vi "RT Main system.vi"   [LabVIEW 2018]
uses:
  <vilib>/FPGAPlugInAG/myRIO-1900/niLvFpga_Open_myRIO-1900.vi
  <vilib>/rvi/interface/common/dynamic/niFpgaDynamicAddResources.vi
  <vilib>/Utility/error.llb/Error Cluster From Error Code.vi
  <vilib>/rvi/errors/niLvFpgaAdjustHostInterfaceError.vi
  <vilib>/FPGAPlugInAG/Dynamic/niLvFpga_Close_Dynamic.vi
  <vilib>/rvi/interface/nirviOpenFPGA/nirviOpenFPGA.xnode
  FPGA Bitfiles/FirstprogramFPGA_FPGATarget_FPGAMain_8XtmiEg1vUo.lvbitx
  FPGA Main.vi
  <vilib>/rvi/interface/nirviReadWriteControl/nirviReadWriteControl.xnode
  <vilib>/rvi/interface/nirviCloseFPGA/nirviCloseFPGA.xnode
  NiFpgaLv.dll
  <vilib>/rvi/interface/Simulation/niFpgaSimulationCallBeginRW.vi
panel:
  # "RT"
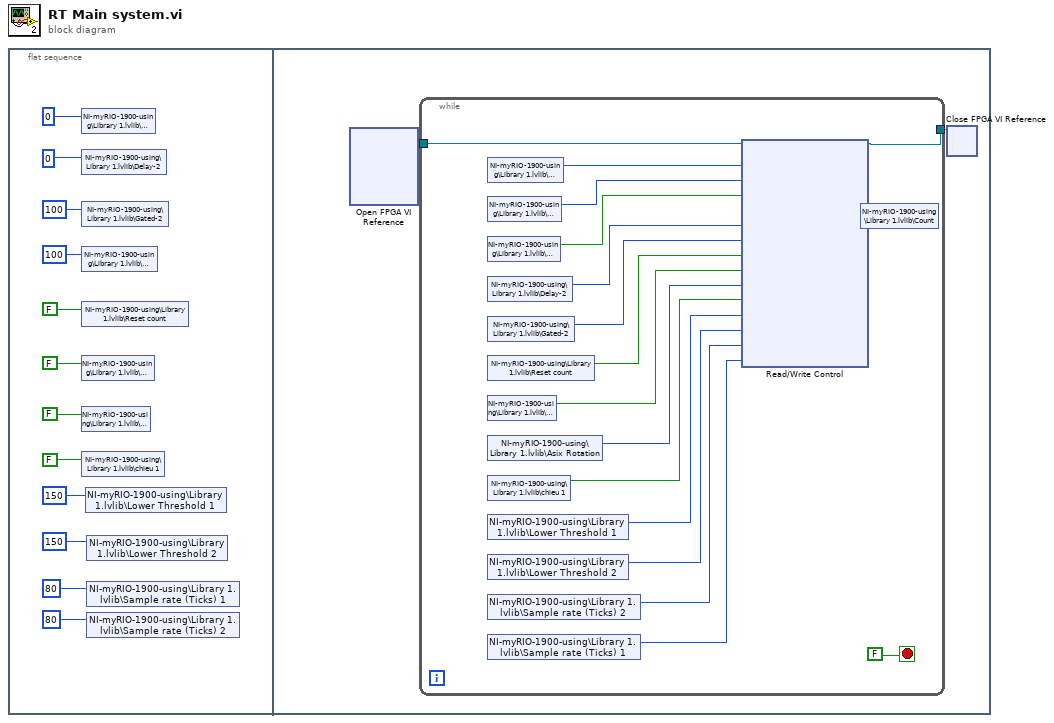
[diagram p0: block diagram]
diagram:
  n1 = flat-sequence {
    frame #0 {
      n2 = shared-variable "NI-myRIO-1900-using\\Library 1.lvlib\\Delay"(i64 0 ("Delay")) -> ()  [unwired: 1 in, 1 out]
      n3 = shared-variable "NI-myRIO-1900-using\\Library 1.lvlib\\Delay-2"(i64 0 ("Delay-2")) -> ()  [unwired: 1 in, 1 out]
      n4 = shared-variable "NI-myRIO-1900-using\\Library 1.lvlib\\Gated-2"(i64 100 ("Gated-2")) -> ()  [unwired: 1 in, 1 out]
      n5 = shared-variable "NI-myRIO-1900-using\\Library 1.lvlib\\Gated"(i64 100 ("Gated")) -> ()  [unwired: 1 in, 1 out]
      n6 = shared-variable "NI-myRIO-1900-using\\Library 1.lvlib\\Reset count"(FALSE ("Reset count")) -> ()  [unwired: 1 in, 1 out]
      n7 = shared-variable "NI-myRIO-1900-using\\Library 1.lvlib\\Reset"(FALSE ("Reset")) -> ()  [unwired: 1 in, 1 out]
      n8 = shared-variable "NI-myRIO-1900-using\\Library 1.lvlib\\Start"(FALSE ("Start")) -> ()  [unwired: 1 in, 1 out]
      n9 = shared-variable "NI-myRIO-1900-using\\Library 1.lvlib\\chieu 1"(FALSE ("chieu 1")) -> ()  [unwired: 1 in, 1 out]
      n10 = shared-variable "NI-myRIO-1900-using\\Library 1.lvlib\\Lower Threshold 1"(i64 150 ("Lower Threshold 1")) -> ()  [unwired: 1 in, 1 out]
      n11 = shared-variable "NI-myRIO-1900-using\\Library 1.lvlib\\Lower Threshold 2"(i64 150 ("Lower Threshold 1")) -> ()  [unwired: 1 in, 1 out]
      n12 = shared-variable "NI-myRIO-1900-using\\Library 1.lvlib\\Sample rate (Ticks) 1"(i64 80 ("Lower Threshold 1")) -> ()  [unwired: 1 in, 1 out]
      n13 = shared-variable "NI-myRIO-1900-using\\Library 1.lvlib\\Sample rate (Ticks) 2"(i64 80 ("Lower Threshold 1")) -> ()  [unwired: 1 in, 1 out]
    }
    frame #1 {
      n14 = xnode "Open FPGA VI Reference"() -> ("FPGA VI Reference Out"=w13:refnum<k20>)  [unwired: 2 in, 1 out]
      n15 = while {
        tunnel: [w30] -> w14
        tunnel: w13 -> [w19]
        stop <- FALSE stop-if-true
        n16 = shared-variable "NI-myRIO-1900-using\\Library 1.lvlib\\Gated"() -> (w29:i64)  [unwired: 1 in, 1 out]
        n17 = shared-variable "NI-myRIO-1900-using\\Library 1.lvlib\\Delay"() -> (w28:i64)  [unwired: 1 in, 1 out]
        n18 = shared-variable "NI-myRIO-1900-using\\Library 1.lvlib\\Reset"() -> (w27:bool)  [unwired: 1 in, 1 out]
        n19 = shared-variable "NI-myRIO-1900-using\\Library 1.lvlib\\Delay-2"() -> (w20:i64)  [unwired: 1 in, 1 out]
        n20 = shared-variable "NI-myRIO-1900-using\\Library 1.lvlib\\Gated-2"() -> (w25:i64)  [unwired: 1 in, 1 out]
        n21 = shared-variable "NI-myRIO-1900-using\\Library 1.lvlib\\Reset count"() -> (w24:bool)  [unwired: 1 in, 1 out]
        n22 = shared-variable "NI-myRIO-1900-using\\Library 1.lvlib\\Start"() -> (w21:bool)  [unwired: 1 in, 1 out]
        n23 = shared-variable "NI-myRIO-1900-using\\Library 1.lvlib\\Asix Rotation"() -> (w23:u64)  [unwired: 1 in, 1 out]
        n24 = shared-variable "NI-myRIO-1900-using\\Library 1.lvlib\\chieu 1"() -> (w22:bool)  [unwired: 1 in, 1 out]
        n25 = shared-variable "NI-myRIO-1900-using\\Library 1.lvlib\\Lower Threshold 1"() -> (w18:i64)  [unwired: 1 in, 1 out]
        n26 = shared-variable "NI-myRIO-1900-using\\Library 1.lvlib\\Lower Threshold 2"() -> (w17:i64)  [unwired: 1 in, 1 out]
        n27 = shared-variable "NI-myRIO-1900-using\\Library 1.lvlib\\Sample rate (Ticks) 2"() -> (w16:i64)  [unwired: 1 in, 1 out]
        n28 = shared-variable "NI-myRIO-1900-using\\Library 1.lvlib\\Sample rate (Ticks) 1"() -> (w15:i64)  [unwired: 1 in, 1 out]
        n29 = xnode "Read/Write Control"("FPGA VI Reference In"=w19, "Gated-1  (ns)"=w29, "Delay-1 (ns)"=w28, "reset"=w27, "Delay-2 (ns)"=w20, "Gated-2  (ns)2"=w25, "reset count"=w24, "start 1"=w21, "Asix Rotation"=w23, "chieu 1"=w22, "Lower Threshold 1"=w18, "Lower Threshold 2"=w17, "Sample rate (Ticks) 2"=w16, "Sample rate (Ticks) 1"=w15) -> ("FPGA VI Reference Out"=w30:refnum<k20>, "Count"=w26:i64)  [unwired: 1 in, 1 out]
        n30 = shared-variable "NI-myRIO-1900-using\\Library 1.lvlib\\Count"(w26) -> ()  [unwired: 1 in, 1 out]
      }
      n31 = xnode "Close FPGA VI Reference"("FPGA VI Reference In"=w14) -> ()  [unwired: 1 in, 1 out]
    }
  }
